vi "SLSC Get Module Name from IP Address_O2.vi"(0 "Chassis IP Address":string="192.168.8.130", 1 "Username":string="admin", 3 "Password":string, 5 "Slot #":u32=6, 11 "Error In":errorcluster, 12 "connect timeout":dbl=50.0) -> (4 "SLSC Module Name":string, 6 "Dev.ProductNum":u32, 8 "Dev.VendorNum":u32, 10 "SLSC Chassis Name":string, 15 "Error Out":errorcluster)   [LabVIEW 2017]
uses:
  <vilib>/nisyscfg/Close (System).vi
  <vilib>/SLSC/Initialize Session with Devices.vi
  <vilib>/SLSC/Initialize Session without Resources.vi
  <vilib>/SLSC/Close Session.vi
  <vilib>/SLSC/SLSC.lvlib
  <resource>/objmgr/slsc.rc
  <vilib>/nisyscfg/nisyscfg.lvlib
  <resource>/objmgr/nisysapi.rc
panel:
  out "concatenated string":string
  out "session out debug":string
  out "Dev.SlotNum":u32
  out "Module Found?":bool
  out "Host Name":string
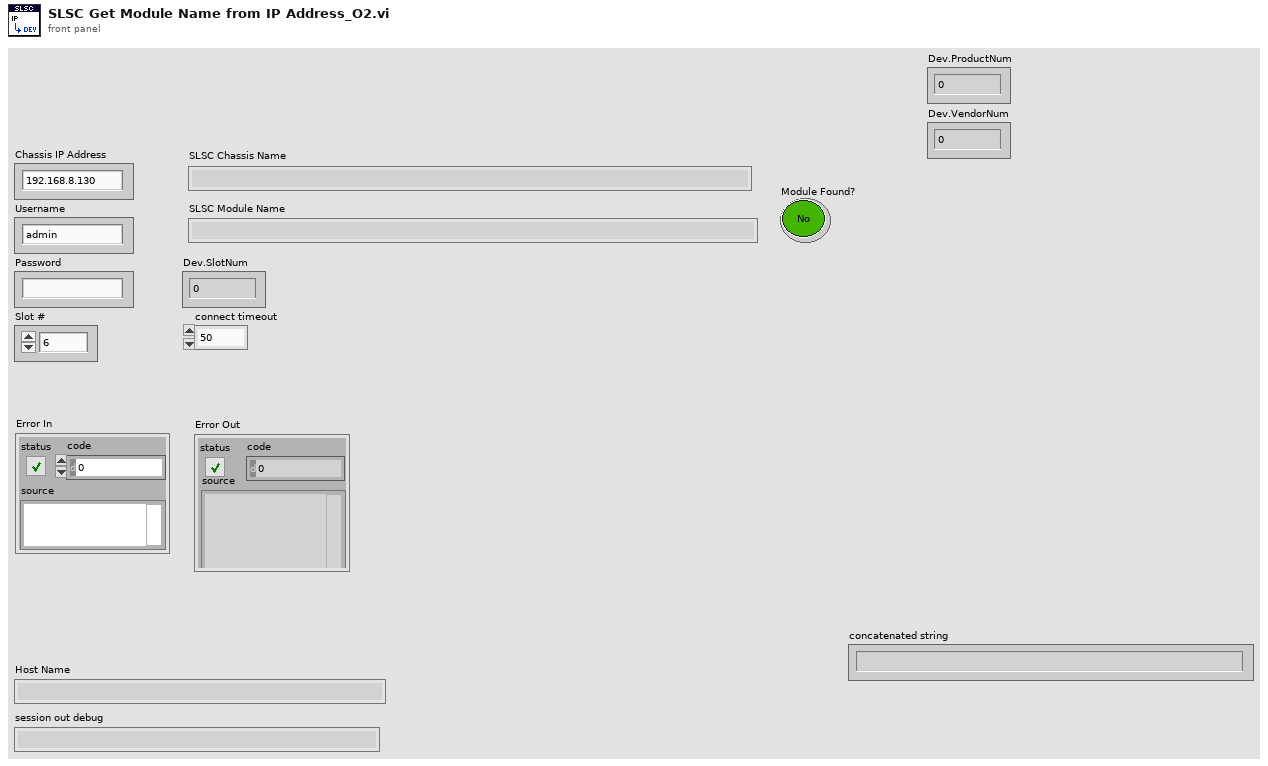
[diagram p1: front panel]
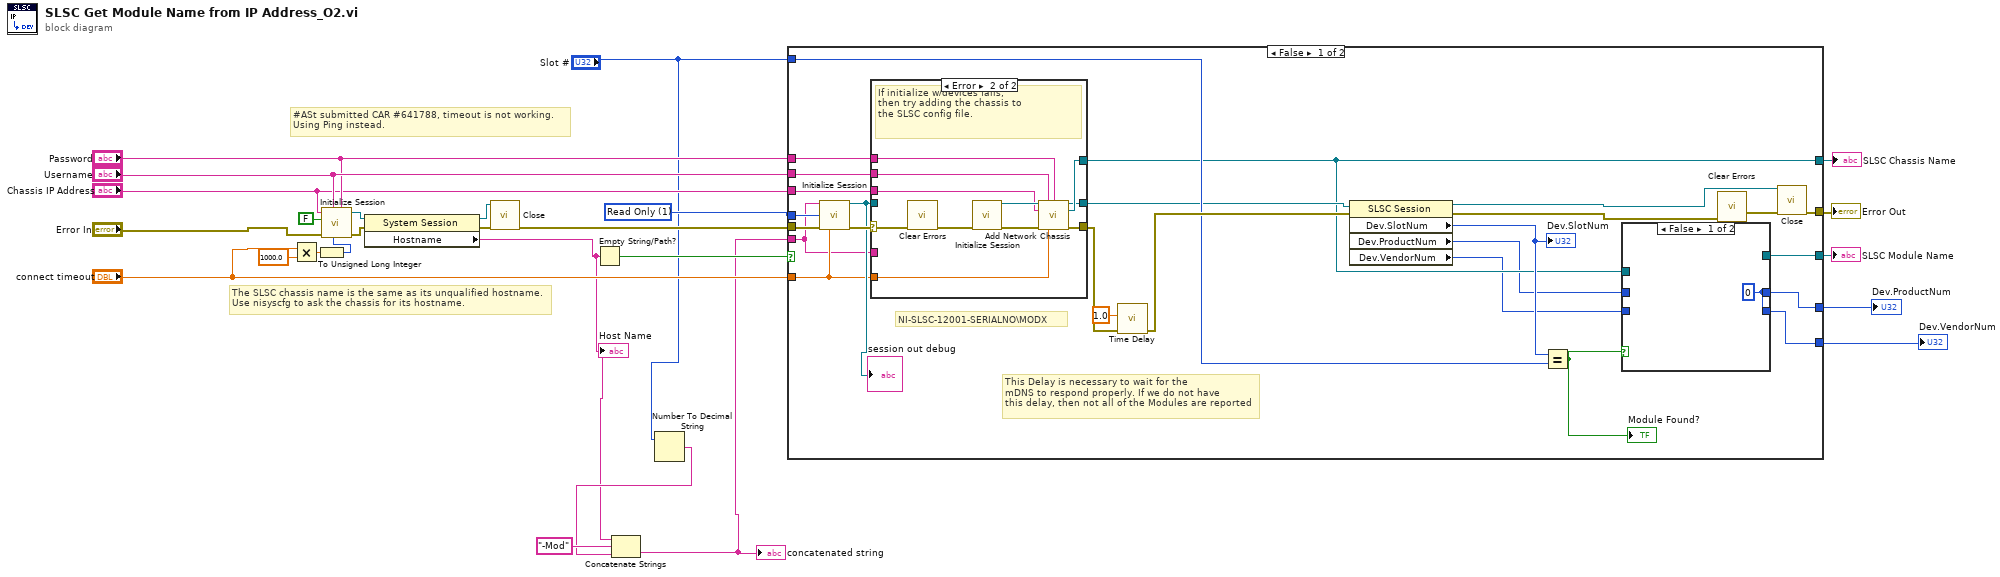
[diagram p0: block diagram]
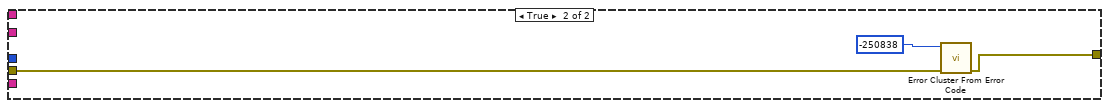
[diagram p4: hidden frame]
diagram:
  w26 = 1 items=["None"=0, "Read Only"=1, "Read/Write"=3] ("reservation access (Read/Write)")
  # "#ASt submitted CAR #641788, timeout is not working.\nUsing Ping instead."
  # "The SLSC chassis name is the same as its unqualified hostname.\nUse nisyscfg to ask the chassis for its hostname."
  n1 = Multiply(x="connect timeout", y=1000.0) -> (x*y=w6:dbl)
  n2 = To Unsigned Long Integer(number=w6) -> (unsigned 32bit integer=w5:u32)
  n3 = call <vilib>:"Initialize Session.vi"("Password"="Password", "Connect Timeout (4000 ms)"=w5, "User Name"="Username", "error in (no error)"="Error In", "Force Property Refresh (T)"=FALSE, "Target (localhost)"="Chassis IP Address") -> ("error out"=w10:errorcluster, "Session out"=w11:refnum<k21>)  [unwired: 4 in]
  n4 = property class="System Session"(reference=w11, error in=w10) -> (reference out=w8:refnum<k21>, error out=w9:errorcluster, "Hostname"=w13:string)
  "Host Name" <- w13
  n5 = call-poly <vilib>:"Close.vi"("error in (no error)"=w9, "Session in"=w8) -> ("error out"=w20:errorcluster)  [unwired: 9 in]
  n6 = Empty String/Path?(string/path=w13) -> (empty?=w23:bool)
  n7 = Number To Decimal String(number="Slot #") -> (decimal integer string=w17:string)  [unwired: 1 in]
  n8 = Concatenate Strings(w13, "-Mod" ("string"), w17) -> (w12:string)
  "concatenated string" <- w12
  n9 = case shown="False" w23 {
    tunnel: [w40 w73] -> w16
    tunnel: w20 -> [w51 w71]
    tunnel: w26 -> [w50 _]
    tunnel: "Chassis IP Address" -> [w47 _]
    tunnel: "Username" -> [w46 _]
    tunnel: "Password" -> [w45 _]
    tunnel: [w32 _] -> w15
    tunnel: "connect timeout" -> [w43 _]
    tunnel: [w42 _] -> w14
    tunnel: w12 -> [w41 _]
    tunnel: "Slot #" -> [w36 _]
    tunnel: [w27 _] -> w2
    tunnel: [w28 _] -> w1
    frame False {
      # "This Delay is necessary to wait for the \nmDNS to respond properly. If we do not have\nthis delay, then not all of the Modules are reported"
      # "NI-SLSC-12001-SERIALNO\\MODX"
      n10 = call-poly <vilib>:"Initialize Session.vi"("devices"=w41, "reservation access (Read/Write)"=w50, "error in (no error)"=w51, "connect timeout (60 sec)"=w43) -> ("session out"=w48:refnum<k21>, "error out"=w49:errorcluster)  [unwired: 10 in]
      "session out debug" <- w48
      n11 = case shown="Error" w49 {
        selector: w49 -> [w59 w70]
        tunnel: [w59 w62] -> w39
        tunnel: [w58 w63] -> w33
        tunnel: w48 -> [w58 _]
        tunnel: w47 -> [_ w68]
        tunnel: w46 -> [_ w66]
        tunnel: w45 -> [_ w65]
        tunnel: [w57 w64] -> w32
        tunnel: w41 -> [w57 _]
        tunnel: w43 -> [_ w60]
        frame No Error {
          # "If initialize w/devices succeeds,\nthen the SLSC driver already\nknows about this chassis via\nmDNS or the config file."
        }
        frame Error {
          # "If initialize w/devices fails,\nthen try adding the chassis to\nthe SLSC config file."
          n12 = call <vilib>:"Clear Errors.vi"("error in (no error)"=w70) -> ("error out"=w61:errorcluster)  [unwired: 5 in, 1 out]
          n13 = call-poly <vilib>:"Initialize Session.vi"("error in (no error)"=w61) -> ("session out"=w69:refnum<k21>, "error out"=w67:errorcluster)  [unwired: 13 in]
          n14 = call <vilib>:"Add Network Chassis.vi"("session in"=w69, "username"=w66, "password"=w65, "chassis IP address/hostname"=w68, "error in (no error)"=w67, "connect timeout (60 sec)"=w60) -> ("session out"=w63:refnum<k21>, "chassis out"=w64:refnum<k21>, "error out"=w62:errorcluster)  [unwired: 7 in]
        }
      }
      n15 = call "Time Delay"("error in (no error)"=w39, "Delay Time (s)"=1.0) -> ("error out"=w38:errorcluster)  [unwired: 9 in]
      n16 = property class="SLSC Session"(reference=w33, error in=w38) -> (reference out=w52:refnum<k21>, error out=w44:errorcluster, "Dev.SlotNum"=w34:u32, "Dev.ProductNum"=w30:u32, "Dev.VendorNum"=w29:u32)
      "Dev.SlotNum" <- w34
      n17 = Equal?(x=w34, y=w36) -> (x = y?=w35:bool)
      "Module Found?" <- w35
      n18 = case shown="False" w35 {
        tunnel: w32 -> [_ w56]
        tunnel: [_ w56] -> w42
        tunnel: w30 -> [_ w55]
        tunnel: w29 -> [_ w54]
        tunnel: [w53 w55] -> w28
        tunnel: [w53 w54] -> w27
        frame False {
          w53 = u32 0 ("Dev.ProductNum")
        }
        frame True {
        }
      }
      n19 = call <vilib>:"Clear Errors.vi"("error in (no error)"=w44) -> ("error out"=w31:errorcluster)  [unwired: 5 in, 1 out]
      n20 = call-poly <vilib>:"Close.vi"("session in"=w52, "error in (no error)"=w31) -> ("error out"=w40:errorcluster)  [unwired: 13 in]
    }
    frame True {
      n21 = call <vilib>:"Error Cluster From Error Code.vi"("error in (no error)"=w71, "error code (0)"=-250838 ("code")) -> ("error out"=w73:errorcluster)  [unwired: 7 in]
    }
  }
  "SLSC Chassis Name" <- w15
  "Error Out" <- w16
  "SLSC Module Name" <- w14
  "Dev.VendorNum" <- w2
  "Dev.ProductNum" <- w1
